vi "Max Bin Read.vi"(1 "FPGA VI Reference In":refnum<k20>, 4 "error in":errorcluster) -> (14 "Max Bin":i32, 15 "Max Amp":fxp<+,46,22>, 16 "Next Bin":i32, 17 "Next Amp":fxp<+,46,22>, 18 "Prev Bin":i32, 19 "Prev Amp":fxp<+,46,22>)   [LabVIEW 2014]
uses:
  <vilib>/Utility/error.llb/Error Cluster From Error Code.vi
  <vilib>/rvi/errors/niLvFpgaAdjustHostInterfaceError.vi
  <vilib>/rvi/interface/nirviMethod/nirviMethod.xnode
  <vilib>/FPGAPlugInAG/Dynamic/niLvFpga_ReadFifo_Dynamic.vi
  <vilib>/rvi/errors/niLvFpgaMergeErrorWithErrorCode.vi
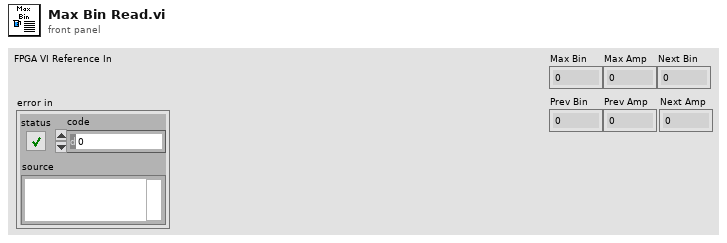
[diagram p1: front panel]
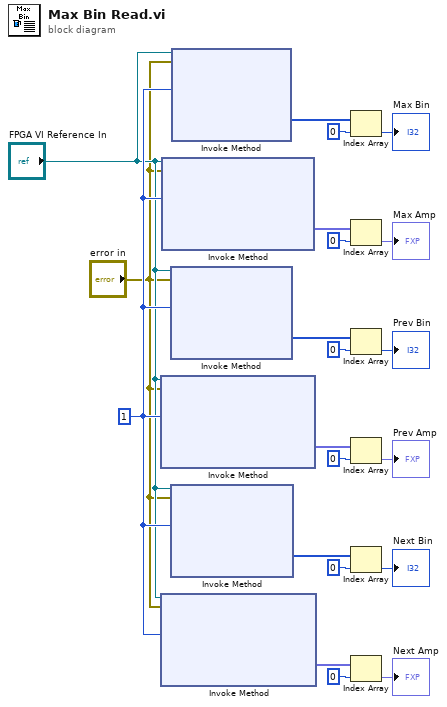
[diagram p0: block diagram]
diagram:
  w21 = u32 1 ("Number of Elements")
  n1 = xnode "Invoke Method"("FPGA VI Reference In"="FPGA VI Reference In", "error in"="error in", "Number of Elements"=w21) -> ("Data"=w12:fxp<+,46,22>[])  [unwired: 1 in, 3 out]
  n2 = xnode "Invoke Method"("FPGA VI Reference In"="FPGA VI Reference In", "error in"="error in", "Number of Elements"=w21) -> ("Data"=w4:fxp<+,46,22>[])  [unwired: 1 in, 3 out]
  n3 = xnode "Invoke Method"("FPGA VI Reference In"="FPGA VI Reference In", "error in"="error in", "Number of Elements"=w21) -> ("Data"=w16:fxp<+,46,22>[])  [unwired: 1 in, 3 out]
  n4 = xnode "Invoke Method"("FPGA VI Reference In"="FPGA VI Reference In", "error in"="error in", "Number of Elements"=w21) -> ("Data"=w14:i32[])  [unwired: 1 in, 3 out]
  n5 = xnode "Invoke Method"("FPGA VI Reference In"="FPGA VI Reference In", "error in"="error in", "Number of Elements"=w21) -> ("Data"=w7:i32[])  [unwired: 1 in, 3 out]
  n6 = xnode "Invoke Method"("FPGA VI Reference In"="FPGA VI Reference In", "error in"="error in", "Number of Elements"=w21) -> ("Data"=w20:i32[])  [unwired: 1 in, 3 out]
  n7 = Index Array(array=w20, index=0) -> (element=→"Max Bin":i32)
  n8 = Index Array(array=w16, index=0) -> (element=→"Max Amp":fxp<+,46,22>)
  n9 = Index Array(array=w14, index=0) -> (element=→"Prev Bin":i32)
  n10 = Index Array(array=w12, index=0) -> (element=→"Prev Amp":fxp<+,46,22>)
  n11 = Index Array(array=w7, index=0) -> (element=→"Next Bin":i32)
  n12 = Index Array(array=w4, index=0) -> (element=→"Next Amp":fxp<+,46,22>)
